vi "Z_Read_Data.vi"(8 "error in":errorcluster, 10 "IN":dbl, 11 "VISA Refnum in":refnum<visa-resource-name>) -> (0 "error out":errorcluster, 2 "OUT":dbl, 3 "VISA Refnum out":refnum<visa-resource-name>)   [LabVIEW 2018]
doc: "Processes any returned data from a connected Hokuyo URG-04LX-UG01 device and returns an array of distance measurements in millimeters via the <b>Distance Measurements</b> indicator."
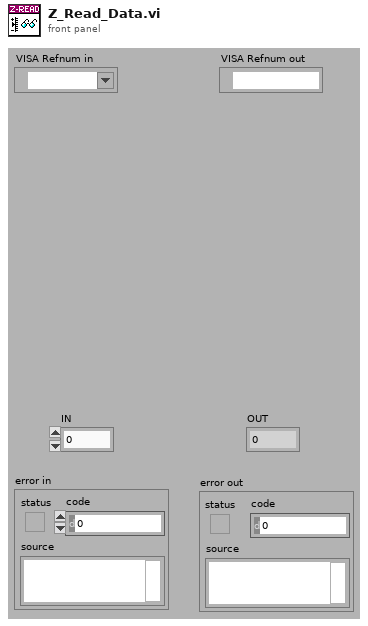
[diagram p1: front panel]
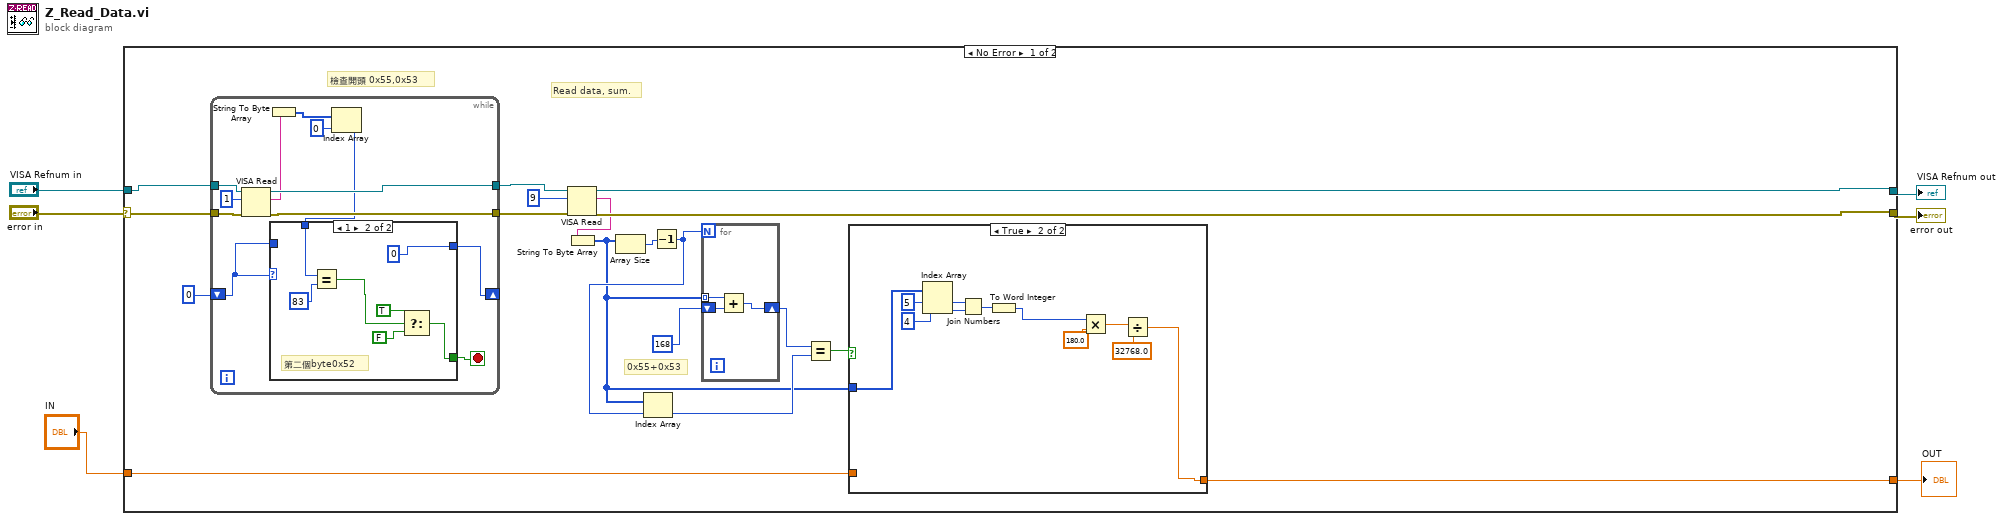
[diagram p0: block diagram]
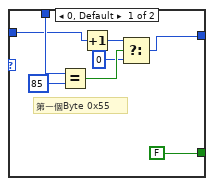
[diagram p3: hidden frame]
diagram:
  n1 = case shown="No Error" "error in" {
    selector: "error in" -> [w22 w69]
    tunnel: [w18 w69] -> w6
    tunnel: [w17 w68] -> w5
    tunnel: "VISA Refnum in" -> [w23 w68]
    tunnel: "IN" -> [w8 w67]
    tunnel: [w7 w67] -> w1
    frame No Error {
      # "0x55+0x53"
      # "檢查開頭 0x55,0x53"
      # "Read data, sum."
      n2 = while {
        tunnel: w23 -> [w51]
        tunnel: [w49] -> w21
        tunnel: w22 -> [w50]
        tunnel: [w48] -> w20
        shift-right: [w46] -> _
        shift-left: 0 -> [w45]
        stop <- w40 stop-if-true
        n3 = VISA Read(VISA resource name=w51, byte count=u32 1, error in (no error)=w50) -> (VISA resource name out=w49:refnum<visa-resource-name>, read buffer=w44:string, error out=w48:errorcluster)  [unwired: 1 out]
        n4 = String To Byte Array(string=w44) -> (unsigned byte array=w43:u8[])
        n5 = Index Array(array=w43, index=0) -> (element=w41:u8)
        n6 = case shown="1" w45 {
          tunnel: [w56 0 ("f")] -> w46
          tunnel: w45 -> [w55 _]
          tunnel: w41 -> [w59 w66]
          tunnel: [FALSE w61] -> w40
          frame 0, Default {
            # "第一個Byte 0x55"
            n7 = Equal?(x=w59, y=u8 85) -> (x = y?=w54:bool)
            n8 = Increment(x=w55) -> (x+1=w57:i32)
            n9 = Select(t=w57, s=w54, f=0) -> (s? t:f=w56:i32)
          }
          frame 1 {
            # "第二個byte0x52"
            n10 = Equal?(x=w66, y=u8 83) -> (x = y?=w62:bool)
            n11 = Select(t=TRUE, s=w62, f=FALSE) -> (s? t:f=w61:bool)
          }
        }
      }
      n12 = VISA Read(VISA resource name=w21, byte count=u32 9, error in (no error)=w20) -> (VISA resource name out=w17:refnum<visa-resource-name>, read buffer=w16:string, error out=w18:errorcluster)  [unwired: 1 out]
      n13 = String To Byte Array(string=w16) -> (unsigned byte array=w9:u8[])
      n14 = Array Size(array=w9) -> (size(s)=w15:i32)
      n15 = Decrement(x=w15) -> (x-1=w11:i32)
      n16 = Index Array(array=w9, index=w11) -> (element=w10:u8)
      n17 = for {
        N: w11 -> [_]
        tunnel: w9 -> [w39] mode=indexing
        shift-right: [w37] -> w12
        shift-left: u8 168 -> [w38]
        n18 = Add(x=w39, y=w38) -> (x+y=w37:u8)
      }
      n19 = Equal?(x=w12, y=w10) -> (x = y?=w13:bool)
      n20 = case shown="True" w13 {
        tunnel: w9 -> [_ w36]
        tunnel: w8 -> [w25 _]
        tunnel: [w25 w26] -> w7
        frame False {
        }
        frame True {
          n21 = Index Array(array=w36, index #1=5 ("index"), index #2=4 ("index")) -> (element #1=w30:u8, element #2=w29:u8)
          n22 = Join Numbers(hi=w30, lo=w29) -> ((hi.lo)=w28:u16)
          n23 = To Word Integer(number=w28) -> (16bit integer=w27:i16)
          n24 = Multiply(x=w27, y=180.0) -> (x*y=w32:dbl)
          n25 = Divide(x=w32, y=32768.0) -> (x/y=w26:dbl)
        }
      }
    }
    frame Error {
    }
  }
  "error out" <- w6
  "VISA Refnum out" <- w5
  "OUT" <- w1
